vi "ArmGetRLEOnTarget.vi"() -> (0 "RLEOnTarget":bool)   [LabVIEW 2020]
doc: "Getter for RLEOnTarget\nOutputs:\n--RLEOnTarget--Boolean--"
uses:
  ArmGlobal.vi
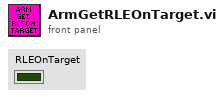
[diagram p1: front panel]
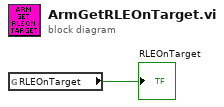
[diagram p0: block diagram]
diagram:
  n1 = global read "ArmGlobal.vi" "RLEOnTarget"() -> (→"RLEOnTarget":bool)
